vi "GlobIndSw1.vi"() -> ()   [LabVIEW 2020]
panel:
  in  "Median Filter Rank":i32=25
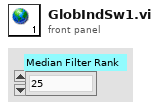
[diagram p1: front panel]
diagram:
